vi "GetSetProgramIntervalString.vi"(0 "VISA resource name":refnum<visa-resource-name>, 1 "get/set":T6=enum."set", 2 "Interval Number (Interval 0 is special case)":i16 min=0 max=300 step=1, 3 "Aux Cluster":T2 {"Group 2 Aux code input" min=0 max=255 step=1; "Group 1 Aux code input" min=0 max=255 step=1}, 4 "Interval Parameters Cluster\n(only first four values are\nused for Interval 0)":T5={"Final Value 1"=0.0, "Final Value 2"=0.0, "Final Value 3"=0.0, "Final Value 4"=0.0, "Deviation 1"=0.0, "Deviation 2"=0.0, "Deviation 3"=0.0, "Deviation 4"=0.0, "hours"=0, "minutes"=0, "seconds"=0, "Parameter Group"=1, "Number Of Loops"=1, "Next Interval"=0} {"Next Interval" min=0 max=300 step=1; "Number Of Loops" min=0 max=9999 step=1; "Parameter Group" min=1 max=4 step=1; "seconds" min=0 max=99 step=1; "minutes" min=0 max=99 step=1; "hours" min=0 max=99 step=1}, 5 "error in":errorcluster, 6 "Active Channels Cluster ( only used for Interval 0)":T4 {"Active Channels code input" min=0 max=15 step=1}, 7 "Options":u16(ring)=1 items=["Product temperature control"=1, "Humidity system"=2, "Low humidity system"=4, "GSoak"=8, "Purge"=16, "Cascade refrigeration"=32, "Power Save mode"=64, "Single-stage refrigeration"=128, "Altitude"=512, "Mechanical boost"=1024, "Product dew point control"=32768]) -> (14 "VISA resource name out":refnum<visa-resource-name>, 15 "8800 Response":string, 19 "error out":errorcluster)   [LabVIEW 2023, in "Thermotron 8800.lvlib"]
doc: "INTV\nCommand name: Send or load program interval string\nCommand type: Programming\nDescription: The query command asks for the interval string that initializes the program (INTV0) or\nfor one of the program intervals (INTVn). During load program by value operations,\nsend an INTV0? command, followed by an INTVn? command for every interval in your\nprogram. Use the PROGn? command to determine how many intervals you need to\nreceive. The operation command sends an interval string to initialize the program\n(INTV0) or one of the program intervals (INTVn).\nInterval 0 syntax: INTV0? or INTV0,fv1,fv2,fv3,fv4,active channels\nWhere:\nfv1 ... fv4 = decimal values for the channel 1 through channel 4 initial values.\nNOTE: The final values of interval 0 are the initial values of interval 1.\nactive channels = two-digit coded integer that assigns the active channels the\nfollowing weight:\n1 = Channel 1\n2 = Channel 2 \n4 = Channel 3 \n8 = Channel 4\n\nInterval n syntax: INTVn? or INTVn,fv1,fv2,fv3,fv4,dv1,dv2,dv3,dv4,hh:mm:ss,pgrp,lp,ni,ax1, ax2,display status,options\nWhere:\nn = interval number\nfv1 ... fv4 = decimal values for the channel 1 through channel 4 final values\ndv1 ... dv4 = decimal values for the channel 1 through channel 4 deviations from set\npoint\nhh:mm:ss = hours (0 to 99), minutes (0 to 99), and seconds (0 to 99). For the time\nfield entry variations, see the TLFT command.\npgrp = parameter group (1 through 4)\nlp = number of loops (0 to 9999)\nni = next interval (1 to 300)\nax1, ax2 = auxiliaries enabled in each AUX group. Auxiliary group 1 refers to\nauxiliaries 1 through 8 and auxiliary group 2 refers to auxiliaries 9 through 16. Each\nvalue is a three-digit coded integer with the following values:\n1 AUX 1 \n2 AUX 2 \n4 AUX 3 \n8 AUX 4 \n16 AUX 5\n32 AUX 6\n64 AUX 7\n128 AUX 8\ndisplay status byte = not used\noptions = The options bytes for the program (0 to 65535). These bytes turn the\noptions on or off. You must turn on the option in order to use its programmed values.\nFor example, to use product temperature control (PTC), you must program the PTC\nchannel and turn the PTC option on. These bytes assign the following weighting\nvalues to the options:\n1 Product temperature control\n2 Humidity system (NOTE: NEVER assign a PTC channel with a humidity\nchannel.)\n4 Low humidity system\n8 GSoak\n16 Purge\n32 Cascade refrigeration (SE-Series chambers only)\n64 Power Save mode (if SE-Series; otherwise sets cascade mode)\n128 Single-stage refrigeration (SE-Series only)\n512 Altitude\n1024 Mechanical boost\n32768 Product dew point control\nData type: Coded integer\nQuery example 1: INTV0?\n8800 response: 30.0, 50.0, 0.0, 0.0,3 (Channel 1 is set to +30 units and channel 2 is set to +50 units; channels 1 and 2 are active.)\nQuery example 2: INTV22?\n8800 response: 52,-67,,,3,10,,,1:10:00,3,5,18,14,26,55,49\nInterval 22 is programmed as follows:\nFinal values: Channel 1 = -52 units, channel 2 = -67 units\nDeviations: Channel 1 = 3 units, channel 2 = 10 units\nTime: 1 hour, 10 minutes\nParameter group: 3\nNumber of loops: 5\nNext interval: 18\nAuxiliaries enabled: AUX 1-2, AUX 1-3, AUX 1-4, AUX 2-2, AUX 2-4, and AUX 2-5\nDisplay status enabled: Looping, auxiliaries, deviations, channel 1, channel 2\nOptions enabled: PTC, purge, cascade refrigeration. NOTE: The commas are left in\nany unused parameter locations to maintain the proper parameter positions in the\nstring\nOperation example 1: INTV0,-10,20,,,3\n8800 response: The 8800 loads the program with a channel 1 initial value of -10 units, a channel 2 value of 20 units, and sets channels 1 and 2 as active.\nOperation example 2: INTV35,75,98,,,5,8,,,0:20:00,1,20,15,3,1,55,150\n8800 response: The 8800 loads the following values into interval 35:\nFinal values: Channel 1 = 75 units, channel 2 = 98 units\nDeviations: Channel 1 = 5 units, channel 2 = 8 units\nTime: 20 minutes\nParameter group: 1\nNumber of loops: 20\nNext interval: 15\nAuxiliaries enabled: AUX 1-1, AUX 1-2, AUX 2-1\nDisplay status enabled: Looping, auxiliaries, deviations, channel 1, channel 2\nOptions enabled: Humidity, low humidity, purge, single-stage refrigeration"
uses:
  Thermotron 8800.lvlib
  Private/get set.ctl
  Private/ActiveChannels.ctl
  Private/AuxSelection.ctl
panel:
  out "Command string to 8800":string
  # "Press control key for multiple selections"
  # "Select Aux boxes"
  # "Select Aux code"
  # "Press control key for multiple selections"
  # "Select Active Channels box"
  # "Select Active Channels code"
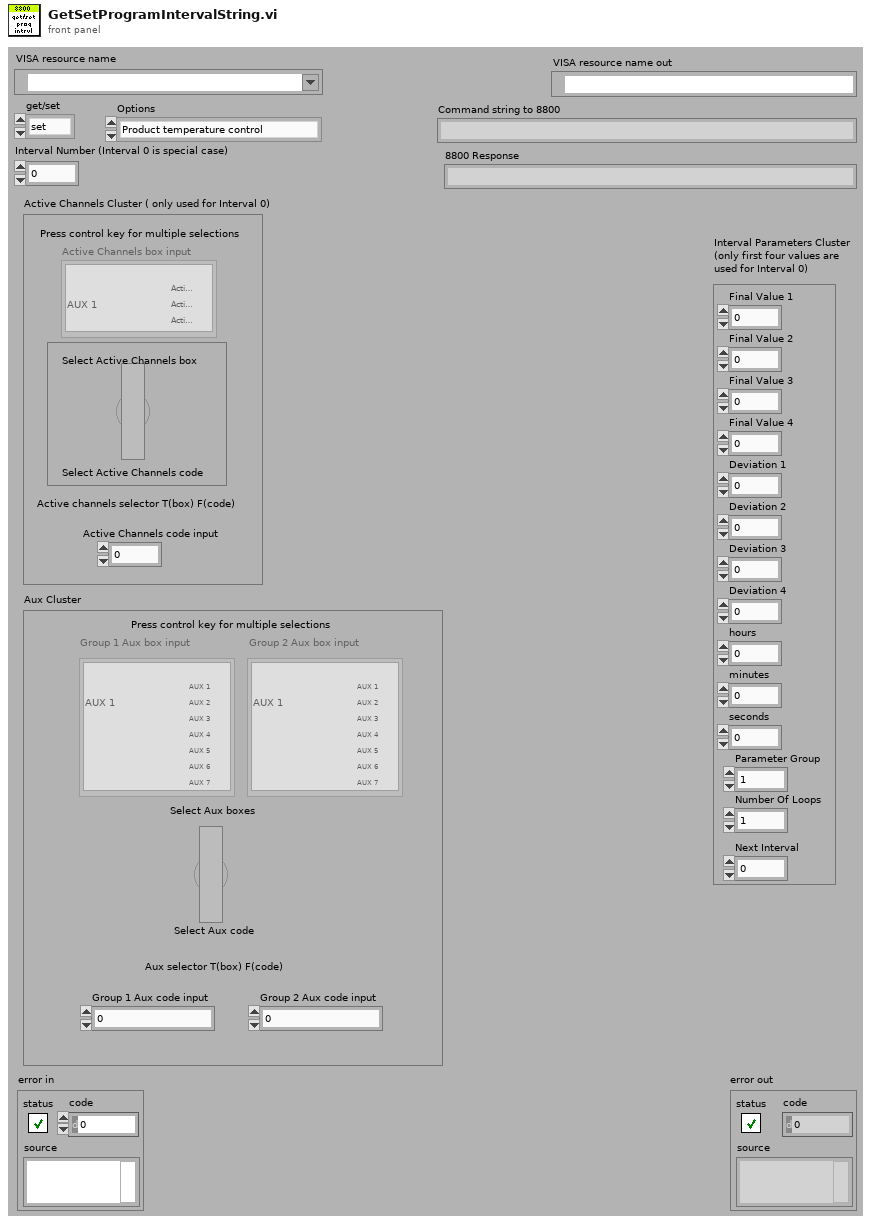
[diagram p1: front panel]
types:
  T1 = typedef "Thermotron 8800.lvlib/AuxSelection.ctl" = i32[]
  T2 = cluster{"Group 1 Aux box input":T1, "Group 2 Aux box input":T1, "Group 1 Aux code input":i32, "Group 2 Aux code input":i32, "Aux selector box":bool}
  T3 = typedef "Thermotron 8800.lvlib/ActiveChannels.ctl" = i32[]
  T4 = cluster{"Active Channels box input":T3, "Active Channels code input":i32, "Active Channels selector T(box) F(code)":bool}
  T5 = cluster{"Final Value 1":sgl, "Final Value 2":sgl, "Final Value 3":sgl, "Final Value 4":sgl, "Deviation 1":sgl, "Deviation 2":sgl, "Deviation 3":sgl, "Deviation 4":sgl, "hours":i8, "minutes":i8, "seconds":i8, "Parameter Group":i8, "Number Of Loops":i16, "Next Interval":i16}
  T6 = typedef "Thermotron 8800.lvlib/get set.ctl" = enum16{"get", "set"}
  T7 = enum8{"Enabled", "Disabled", "Disabled and Grayed Out"}
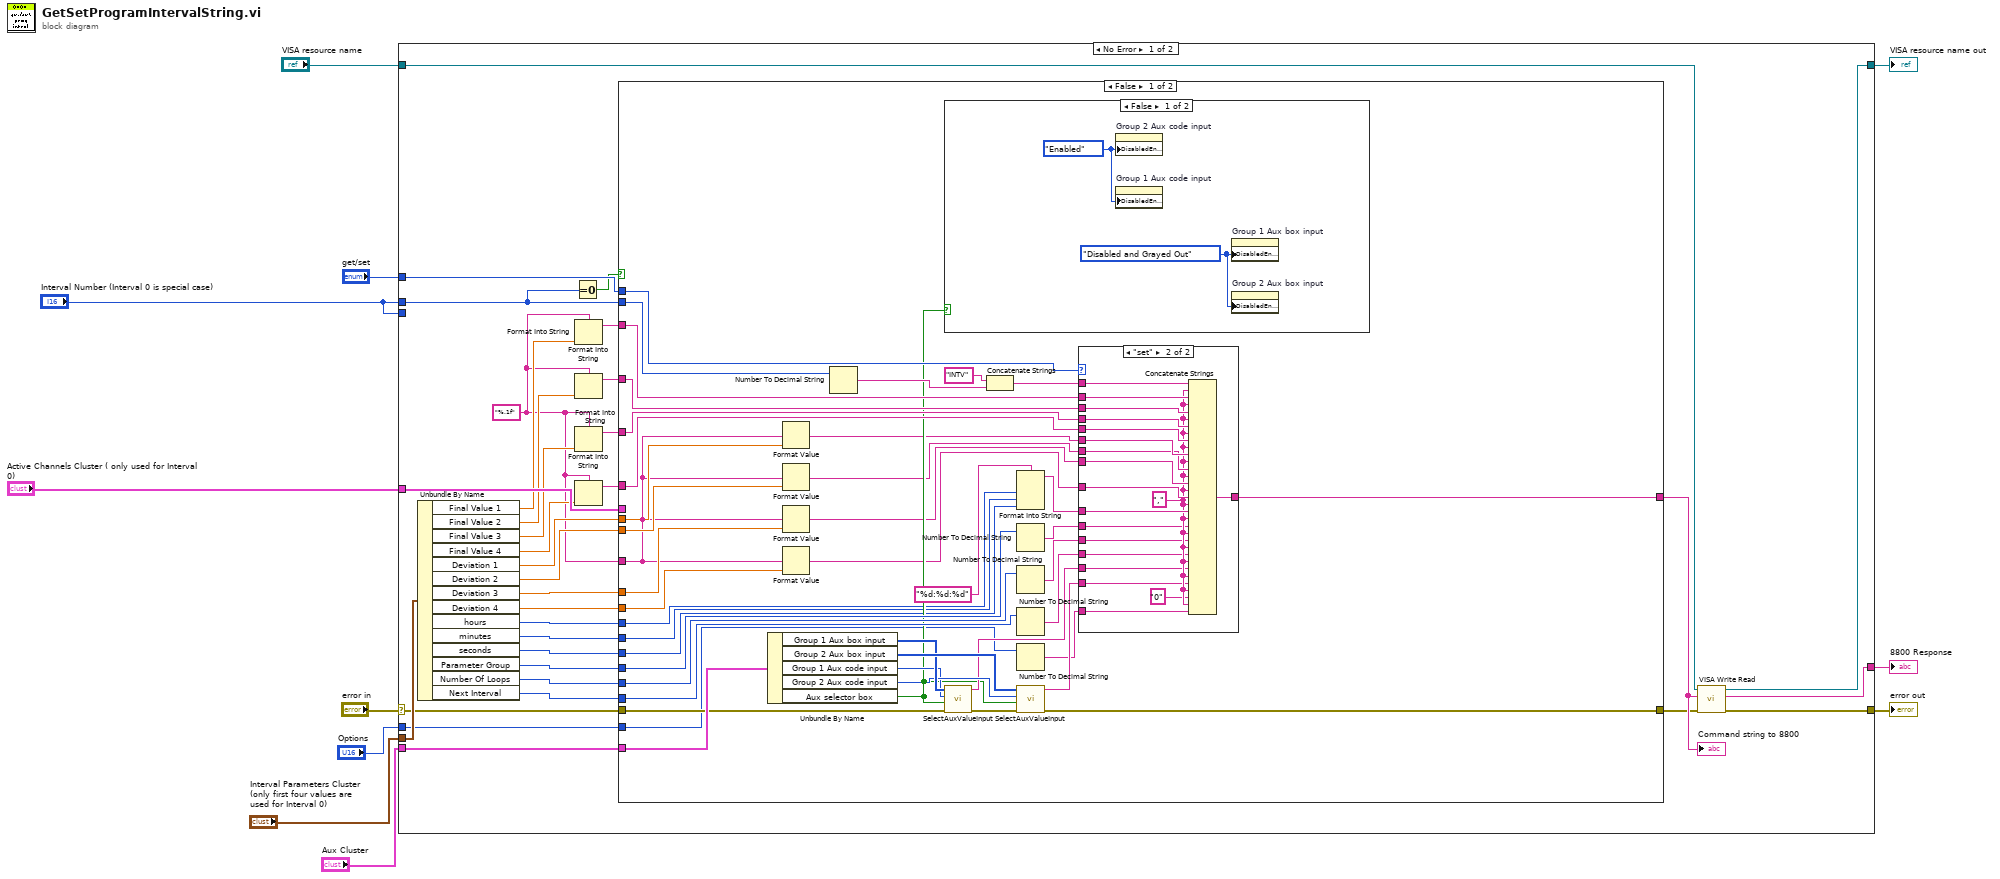
[diagram p0: block diagram]
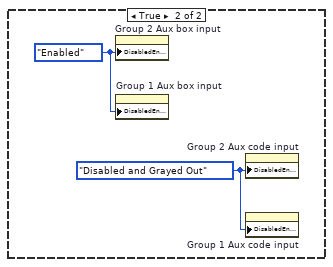
[diagram p2: hidden frame]
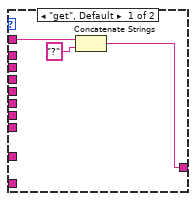
[diagram p3: hidden frame]
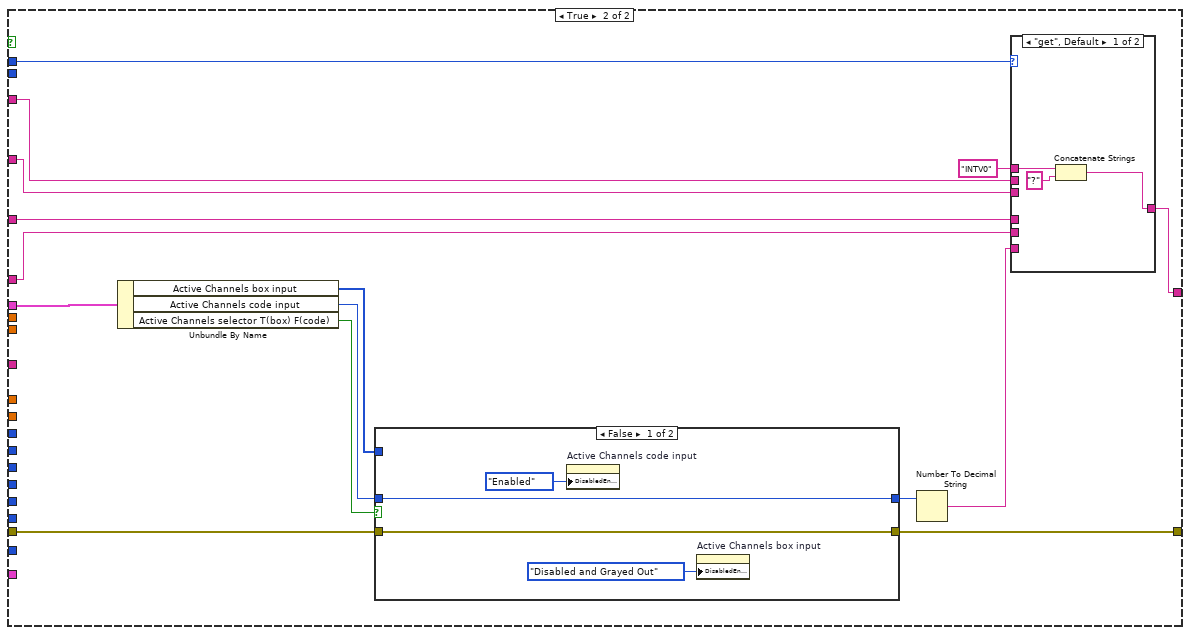
[diagram p4: hidden frame]
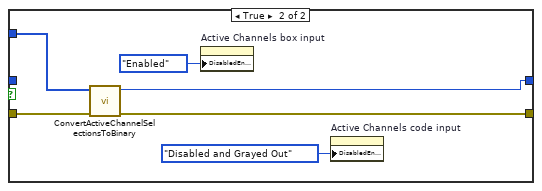
[diagram p5: hidden frame]
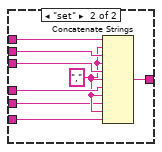
[diagram p6: hidden frame]
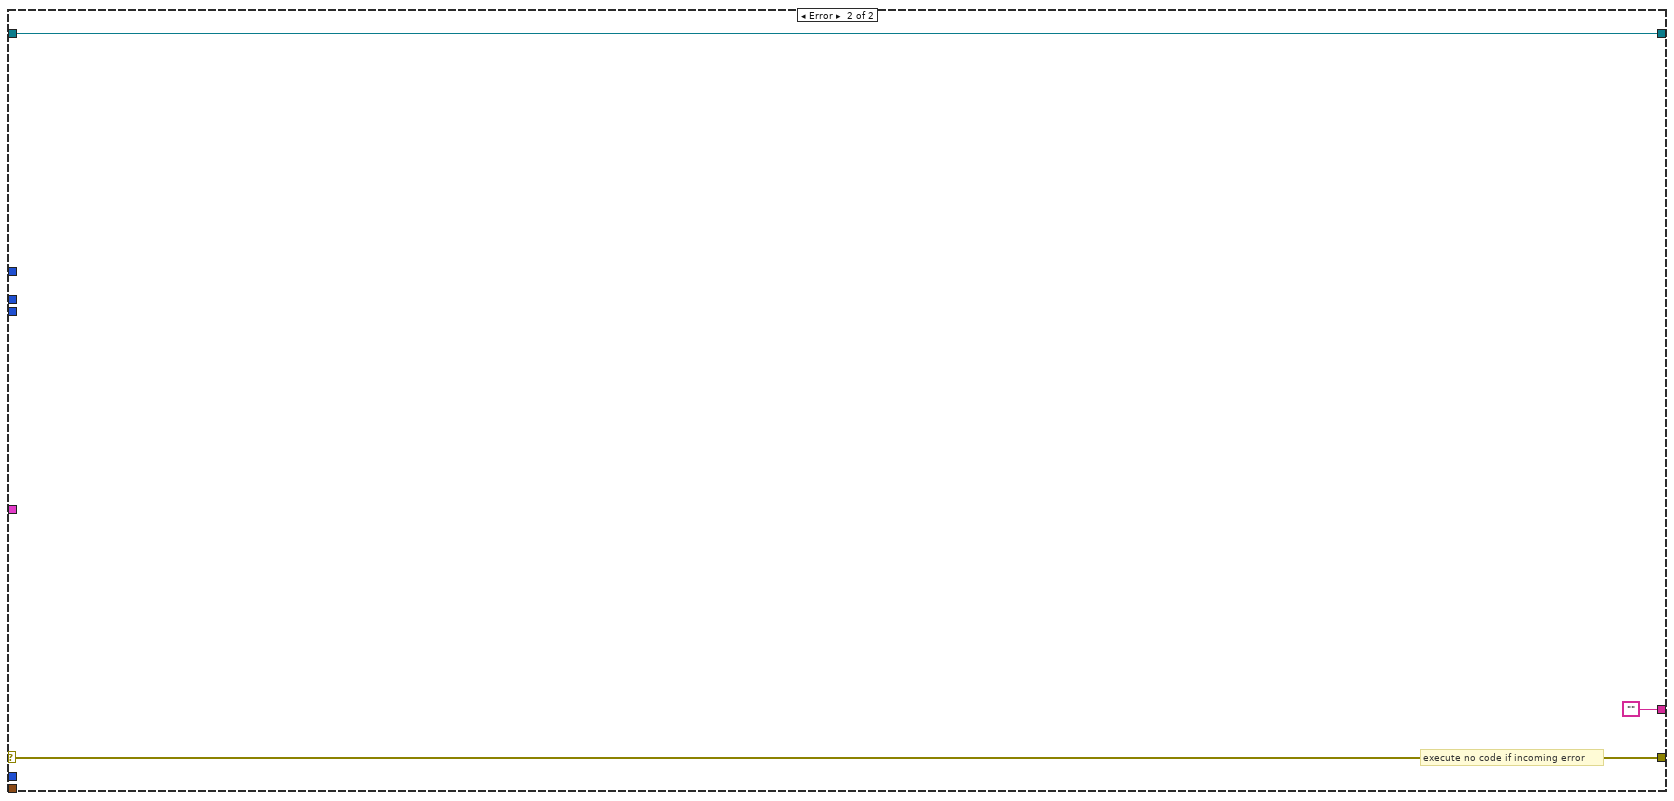
[diagram p7: hidden frame]
diagram:
  n1 = case shown="No Error" "error in" {
    selector: "error in" -> [w22 w152]
    tunnel: [w42 w152] -> w9
    tunnel: [w43 w151] -> w8
    tunnel: "VISA resource name" -> [w44 w151]
    tunnel: [w41 ""] -> w7
    tunnel: "Interval Number (Interval 0 is special case)" -> [_ _]
    tunnel: "get/set" -> [w40 _]
    tunnel: "Interval Number (Interval 0 is special case)" -> [w38 _]
    tunnel: "Interval Parameters Cluster\n(only first four values are\nused for Interval 0)" -> [w37 _]
    tunnel: "Active Channels Cluster ( only used for Interval 0)" -> [w36 _]
    tunnel: "Aux Cluster" -> [w25 _]
    tunnel: "Options" -> [w24 _]
    frame No Error {
      w12 = "%.1f" ("format string")
      n2 = Unbundle By Name(w37) -> ("Final Value 1"=w20:sgl, "Final Value 2"=w18:sgl, "Final Value 3"=w17:sgl, "Final Value 4"=w16:sgl, "Deviation 1"=w35:sgl, "Deviation 2"=w34:sgl, "Deviation 3"=w33:sgl, "Deviation 4"=w32:sgl, "hours"=w31:i8, "minutes"=w30:i8, "seconds"=w29:i8, "Parameter Group"=w28:i8, "Number Of Loops"=w27:i16, "Next Interval"=w26:i16)
      n3 = Equal To 0?(x=w38) -> (x = 0?=w39:bool)
      n4 = Format Into String(format string=w12, w20) -> (resulting string=w19:string)  [unwired: 2 in, 1 out]
      n5 = Format Into String(format string=w12, w18) -> (resulting string=w15:string)  [unwired: 2 in, 1 out]
      n6 = Format Into String(format string=w12, w17) -> (resulting string=w14:string)  [unwired: 2 in, 1 out]
      n7 = Format Into String(format string=w12, w16) -> (resulting string=w13:string)  [unwired: 2 in, 1 out]
      n8 = case shown="False" w39 {
        tunnel: w40 -> [w63 w127]
        tunnel: w38 -> [w81 _]
        tunnel: w19 -> [w80 w126]
        tunnel: w15 -> [w79 w125]
        tunnel: w14 -> [w78 w124]
        tunnel: [w64 w123] -> w23
        tunnel: w36 -> [_ w122]
        tunnel: w35 -> [w56 _]
        tunnel: w34 -> [w59 _]
        tunnel: w33 -> [w54 _]
        tunnel: w32 -> [w53 _]
        tunnel: w31 -> [w48 _]
        tunnel: w30 -> [w47 _]
        tunnel: w29 -> [w46 _]
        tunnel: w28 -> [w87 _]
        tunnel: w27 -> [w86 _]
        tunnel: w26 -> [w85 _]
        tunnel: w13 -> [w77 w116]
        tunnel: w25 -> [w68 _]
        tunnel: w24 -> [w57 _]
        tunnel: w22 -> [w62 w115]
        tunnel: [w61 w114] -> w21
        tunnel: w12 -> [w50 _]
        frame False {
          n9 = Unbundle By Name(w68) -> ("Group 1 Aux box input"=w72:T1, "Group 2 Aux box input"=w73:T1, "Group 1 Aux code input"=w70:i32, "Group 2 Aux code input"=w71:i32, "Aux selector box"=w60:bool)
          n10 = Format Value(format string=w50, value (0)=w56) -> (output string=w55:string)  [unwired: 1 in]
          n11 = Format Value(format string=w50, value (0)=w59) -> (output string=w58:string)  [unwired: 1 in]
          n12 = Format Value(format string=w50, value (0)=w54) -> (output string=w52:string)  [unwired: 1 in]
          n13 = Format Value(format string=w50, value (0)=w53) -> (output string=w51:string)  [unwired: 1 in]
          n14 = Number To Decimal String(number=w81) -> (decimal integer string=w83:string)  [unwired: 1 in]
          n15 = case shown="False" w60 {
            frame False {
              w89 = T7."Disabled and Grayed Out" ("Disabled")
              w88 = T7."Enabled" ("Disabled")
              n16 = property on="Group 2 Aux code input" class="DigNum (strict)"("DisabledEnum"=w88) -> ()  [unwired: 2 in, 2 out]
              n17 = property on="Group 1 Aux code input" class="DigNum (strict)"("DisabledEnum"=w88) -> ()  [unwired: 2 in, 2 out]
              n18 = property on="Group 1 Aux box input" class="LstBox (strict)"("DisabledEnum"=w89) -> ()  [unwired: 2 in, 2 out]
              n19 = property on="Group 2 Aux box input" class="LstBox (strict)"("DisabledEnum"=w89) -> ()  [unwired: 2 in, 2 out]
            }
            frame True {
              w90 = T7."Disabled and Grayed Out" ("Disabled")
              w91 = T7."Enabled" ("Disabled")
              n20 = property on="Group 2 Aux box input" class="LstBox (strict)"("DisabledEnum"=w91) -> ()  [unwired: 2 in, 2 out]
              n21 = property on="Group 1 Aux box input" class="LstBox (strict)"("DisabledEnum"=w91) -> ()  [unwired: 2 in, 2 out]
              n22 = property on="Group 2 Aux code input" class="DigNum (strict)"("DisabledEnum"=w90) -> ()  [unwired: 2 in, 2 out]
              n23 = property on="Group 1 Aux code input" class="DigNum (strict)"("DisabledEnum"=w90) -> ()  [unwired: 2 in, 2 out]
            }
          }
          n24 = call "SelectAuxValueInput.vi"("error in (no error)"=w62, "Aux box input selection"=w60, "Aux code input"=w70, "Aux box input"=w72) -> ("error out"=w69:errorcluster, "aux decimal integer string"=w67:string)  [unwired: 6 in]
          n25 = Concatenate Strings("INTV" ("8800 Command"), w83) -> (w82:string)
          n26 = Format Into String(format string="%d:%d:%d", w48, w47, w46) -> (resulting string=w45:string)  [unwired: 2 in, 1 out]
          n27 = Number To Decimal String(number=w87) -> (decimal integer string=w76:string)  [unwired: 1 in]
          n28 = Number To Decimal String(number=w86) -> (decimal integer string=w75:string)  [unwired: 1 in]
          n29 = Number To Decimal String(number=w85) -> (decimal integer string=w74:string)  [unwired: 1 in]
          n30 = Number To Decimal String(number=w57) -> (decimal integer string=w65:string)  [unwired: 1 in]
          n31 = call "SelectAuxValueInput.vi"("error in (no error)"=w69, "Aux box input selection"=w60, "Aux code input"=w71, "Aux box input"=w73) -> ("error out"=w61:errorcluster, "aux decimal integer string"=w66:string)  [unwired: 6 in]
          n32 = case shown="\"set\"" w63 {
            tunnel: w82 -> [w93 w113]
            tunnel: [w94 w112] -> w64
            tunnel: w80 -> [_ w111]
            tunnel: w79 -> [_ w110]
            tunnel: w78 -> [_ w109]
            tunnel: w77 -> [_ w108]
            tunnel: w55 -> [_ w107]
            tunnel: w58 -> [_ w106]
            tunnel: w52 -> [_ w105]
            tunnel: w51 -> [_ w104]
            tunnel: w45 -> [_ w103]
            tunnel: w76 -> [_ w101]
            tunnel: w75 -> [_ w100]
            tunnel: w74 -> [_ w99]
            tunnel: w67 -> [_ w98]
            tunnel: w66 -> [_ w97]
            tunnel: w65 -> [_ w95]
            frame "get", Default {
              n33 = Concatenate Strings(w93, "?" ("8800 Command")) -> (w94:string)
            }
            frame "set" {
              w102 = "," ("string")
              n34 = Concatenate Strings(w113, w102, w111, w102, w110, w102, w109, w102, w108, w102, w107, w102, w106, w102, w105, w102, w104, w102, w103, w102, w101, w102, w100, w102, w99, w102, w98, w102, w97, w102, "0" ("string"), w102, w95) -> (w112:string)
            }
          }
        }
        frame True {
          n35 = Unbundle By Name(w122) -> ("Active Channels box input"=w120:T3, "Active Channels code input"=w119:i32, "Active Channels selector T(box) F(code)"=w121:bool)
          n36 = case shown="False" w121 {
            tunnel: w120 -> [_ w138]
            tunnel: w119 -> [w132 _]
            tunnel: [w132 w137] -> w118
            tunnel: w115 -> [w131 w136]
            tunnel: [w131 w135] -> w114
            frame False {
              n37 = property on="Active Channels code input" class="DigNum (strict)"("DisabledEnum"=T7."Enabled" ("Disabled")) -> ()  [unwired: 2 in, 2 out]
              n38 = property on="Active Channels box input" class="LstBox (strict)"("DisabledEnum"=T7."Disabled and Grayed Out" ("Disabled")) -> ()  [unwired: 2 in, 2 out]
            }
            frame True {
              n39 = call "ConvertActiveChannelSelectionsToBinary.vi"("error in (no error)"=w136, "Active Channels"=w138) -> ("error out"=w135:errorcluster, "Active Channels"=w137:i32)  [unwired: 8 in]
              n40 = property on="Active Channels box input" class="LstBox (strict)"("DisabledEnum"=T7."Enabled" ("Disabled")) -> ()  [unwired: 2 in, 2 out]
              n41 = property on="Active Channels code input" class="DigNum (strict)"("DisabledEnum"=T7."Disabled and Grayed Out" ("Disabled")) -> ()  [unwired: 2 in, 2 out]
            }
          }
          n42 = Number To Decimal String(number=w118) -> (decimal integer string=w117:string)  [unwired: 1 in]
          n43 = case shown="\"get\", Default" w127 {
            tunnel: "INTV0" ("8800 Command") -> [w140 w149]
            tunnel: [w141 w148] -> w123
            tunnel: w126 -> [_ w147]
            tunnel: w125 -> [_ w146]
            tunnel: w124 -> [_ w145]
            tunnel: w117 -> [_ w143]
            tunnel: w116 -> [_ w142]
            frame "get", Default {
              n44 = Concatenate Strings(w140, "?" ("8800 Command")) -> (w141:string)
            }
            frame "set" {
              w144 = "," ("string")
              n45 = Concatenate Strings(w149, w144, w147, w144, w146, w144, w145, w144, w142, w144, w143) -> (w148:string)
            }
          }
        }
      }
      "Command string to 8800" <- w23
      n46 = call "VISA Write Read.vi"("error in (no error)"=w21, "8800 Command"=w23, "VISA Refnum in"=w44) -> ("error out"=w42:errorcluster, "read buffer"=w41:string, "VISA Refnum out"=w43:refnum<visa-resource-name>)  [unwired: 6 in]
    }
    frame Error {
      # "execute no code if incoming error"
    }
  }
  "VISA resource name out" <- w8
  "error out" <- w9
  "8800 Response" <- w7
